vi "FGGA_Viewer_2.1.vi"() -> ()   [LabVIEW 2012]
uses:
  <vilib>/Utility/tcp.llb/UDP Multicast Read-Only Open.vi
  <vilib>/regexp/Match Regular Expression.xnode
panel:
  in  "Tab Control":enum32{"MAIN_DATA", "MONITORING"}(tab)
  out "FGGA":cluster{dbl, dbl, dbl}(graph)
  out "FGGA_Mon":cluster{dbl, dbl, dbl}(graph)
  out "Running?":bool
  in  "reset x-axis":bool
  out "error out":errorcluster
  in  "stop":bool
  out "data out":string
  in  "name":string="225.0.0.0"
  in  "Port":u16=50005
  # "CONCENTRATIONS ARE NOT ABSOLUTE"
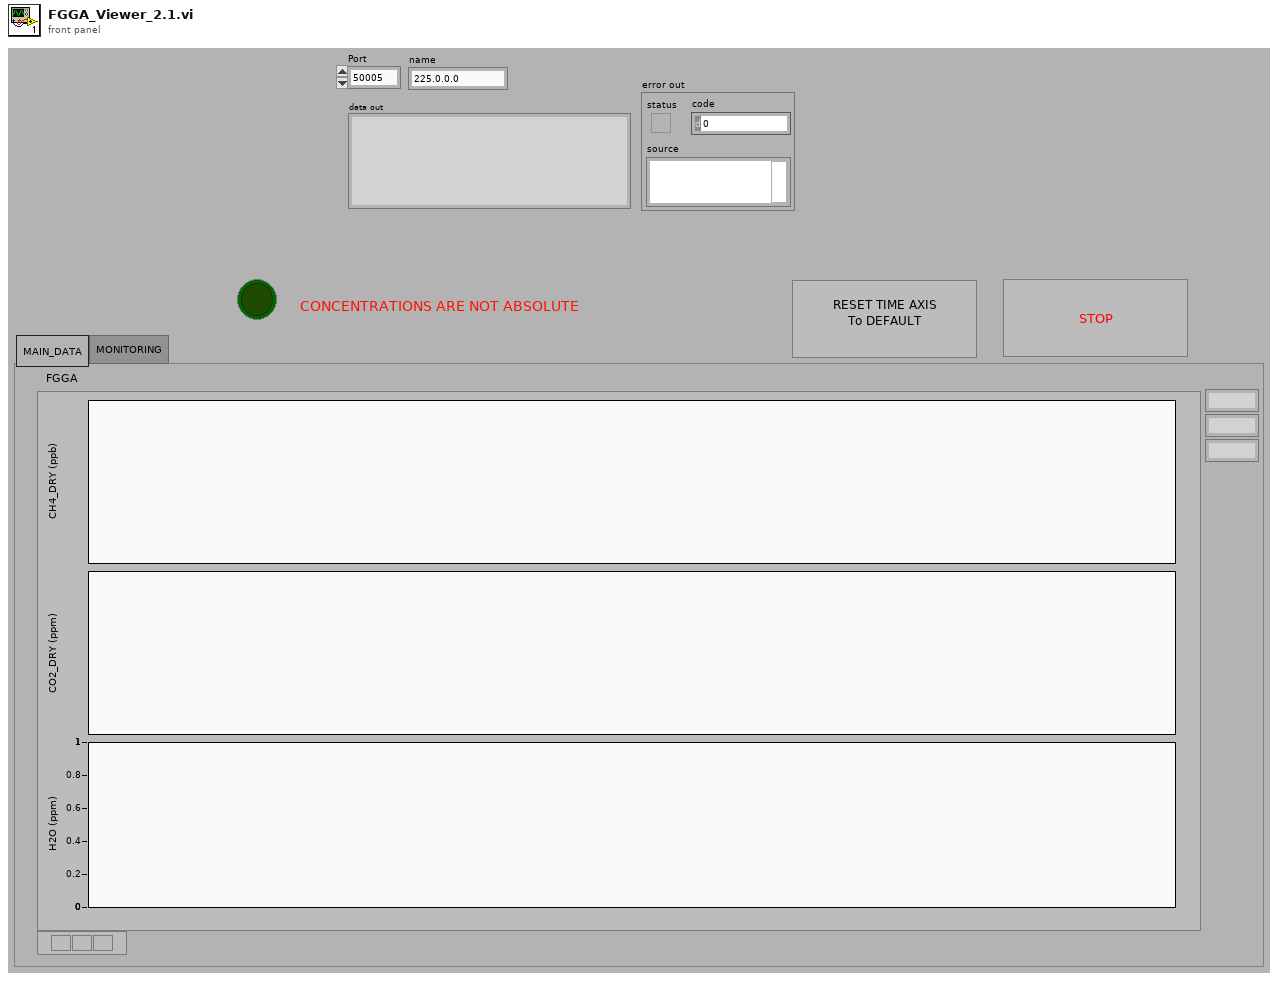
[diagram p1: front panel]
types:
  T1 = cluster{"[0]":i32, "[1]":i32, "[2]":i32, "[3]":i32, "[4]":i32, "[5]":i32, "[6]":i32, "[7]":i32, "[8]":i32}
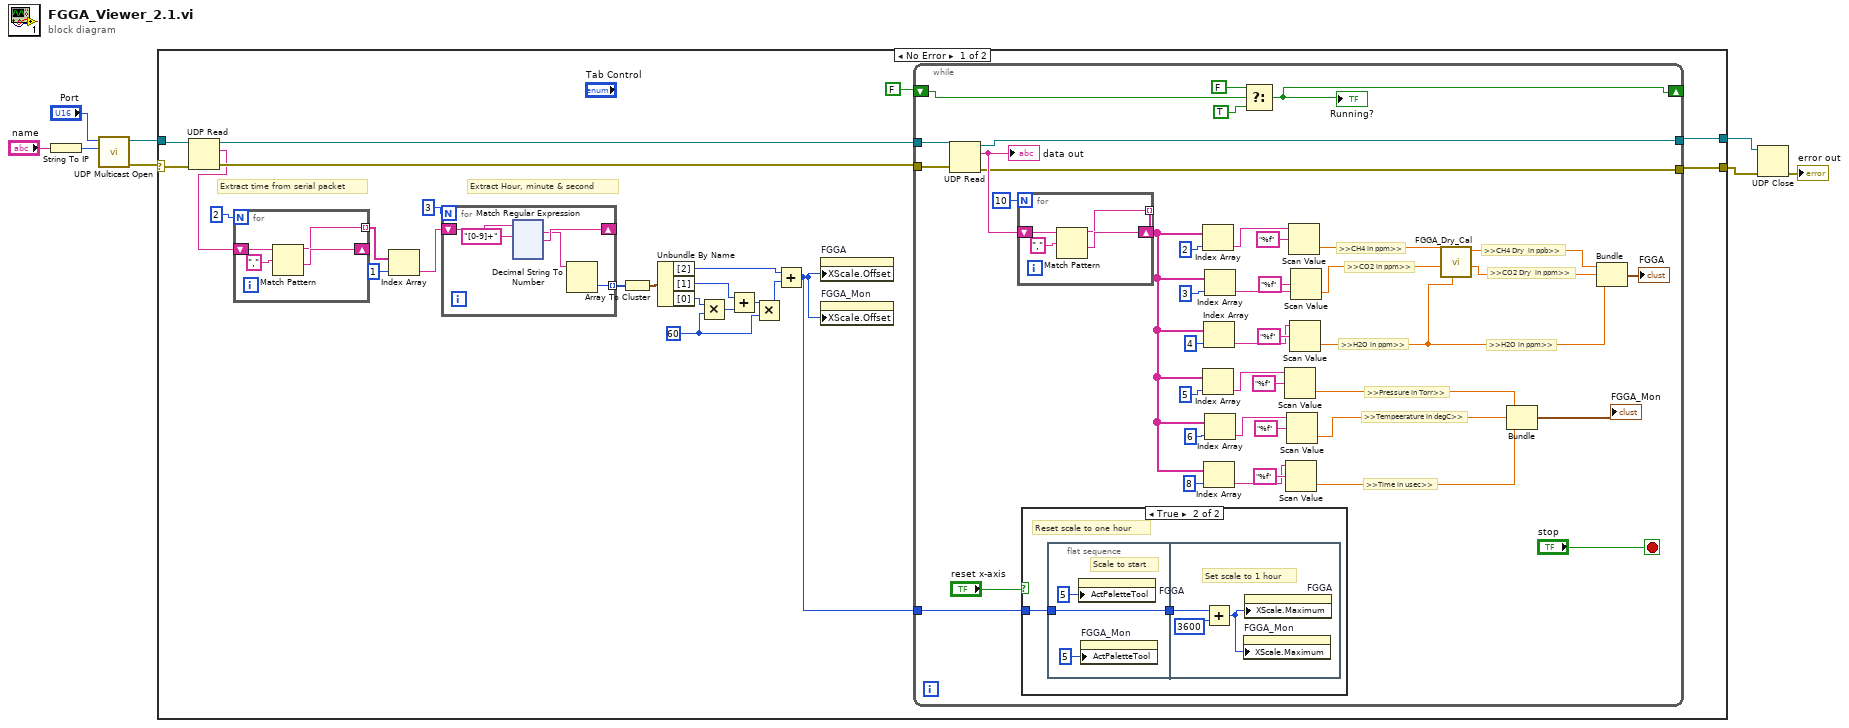
[diagram p0: block diagram]
diagram:
  n1 = String To IP(1:"name") -> (0:w7:u32)
  n2 = call-poly <vilib>:"UDP Multicast Open.vi"("multicast addr"=w7, "port"="Port") -> ("error out"=w4:errorcluster, "connection ID"=w5:refnum<k16>)  [unwired: 7 in, 1 out]
  n3 = case shown="No Error" w4 {
    selector: w4 -> [w29 w206]
    tunnel: w5 -> [w28 w207]
    tunnel: [w31 w206] -> w3
    tunnel: [w30 w207] -> w2
    frame No Error {
      w17 = 60
      # "Extract Hour, minute & second"
      # "Extract time from serial packet"
      n4 = UDP Read(connection ID=w28, 8:w29) -> (data out=w22:string, error out=w26:errorcluster, 3:w27:refnum<k16>)  [unwired: 2 in, 2 out]
      n5 = for {
        N: 2 -> [_]
        shift-right: [w150] -> _
        shift-left: w22 -> [w148]
        tunnel: [w149] -> w23 mode=indexing
        n6 = Match Pattern(string=w148, regular expression=",") -> (before substring=w149:string, after substring=w150:string)  [unwired: 1 in, 2 out]
      }
      n7 = Index Array(array=w23, index=1) -> (element=w18:string)
      n8 = for {
        N: 3 -> [_]
        tunnel: [w33] -> w20 mode=indexing
        shift-right: [w34] -> _
        shift-left: w18 -> [w35]
        n9 = xnode "Match Regular Expression"("input string"=w35, "regular expression"="[0-9]+") -> ("whole match"=w32:string, "after match"=w34:string)  [unwired: 4 in, 3 out]
        n10 = Decimal String To Number(string=w32) -> (number=w33:i32)  [unwired: 2 in, 1 out]
      }
      n11 = Array To Cluster(array=w20) -> (cluster=w19:T1)
      n12 = Unbundle By Name(w19) -> ("[2]"=w11:i32, "[1]"=w12:i32, "[0]"=w13:i32)
      n13 = Multiply(x=w13, y=w17) -> (x*y=w14:i32)
      n14 = Add(x=w12, y=w14) -> (x+y=w15:i32)
      n15 = Multiply(x=w15, y=w17) -> (x*y=w16:i32)
      n16 = Add(x=w11, y=w16) -> (x+y=w9:i32)
      n17 = property on="FGGA" class="WFChart (strict)"("XScale.Offset"=w9) -> ()  [unwired: 2 in, 2 out]
      n18 = property on="FGGA_Mon" class="WFChart (strict)"("XScale.Offset"=w9) -> ()  [unwired: 2 in, 2 out]
      n19 = while {
        tunnel: w27 -> [w193]
        tunnel: w26 -> [w192]
        tunnel: [w180] -> w31
        tunnel: [w178] -> w30
        tunnel: w9 -> [w175]
        shift-right: [w171] -> _
        shift-left: FALSE -> [w174]
        stop <- "stop" stop-if-true
        # ">>H2O in ppm>>"
        # ">>CO2 Dry  in ppm>>"
        # ">>CH4 Dry  in ppb>>"
        # ">>Time in usec>>"
        # ">>Tempeerature in degC>>"
        # ">>Pressure in Torr>>"
        # ">>H2O in ppm>>"
        # ">>CO2 in ppm>>"
        # ">>CH4 in ppm>>"
        n20 = UDP Read(connection ID=w193, 8:w192) -> (data out=w181:string, error out=w180:errorcluster, 3:w178:refnum<k16>)  [unwired: 2 in, 2 out]
        "data out" <- w181
        n21 = for {
          N: 10 -> [_]
          shift-right: [w204] -> _
          shift-left: w181 -> [w202]
          tunnel: [w203] -> w158 mode=indexing
          n22 = Match Pattern(string=w202, regular expression=",") -> (before substring=w203:string, after substring=w204:string)  [unwired: 1 in, 2 out]
        }
        n23 = case shown="True" "reset x-axis" {
          tunnel: w175 -> [_ w195]
          frame False {
          }
          frame True {
            # "Reset scale to one hour"
            n24 = flat-sequence {
              tunnel: w195 -> [w198]
              tunnel: [w198] -> w194
              tunnel: w194 -> [w201]
              frame #0 {
                # "Scale to start"
                n25 = property on="FGGA" class="WFChart (strict)"("ActPaletteTool"=5 ("Palette:Active Tool")) -> ()  [unwired: 2 in, 2 out]
                n26 = property on="FGGA_Mon" class="WFChart (strict)"("ActPaletteTool"=5 ("Palette:Active Tool")) -> ()  [unwired: 2 in, 2 out]
              }
              frame #1 {
                # "Set scale to 1 hour"
                n27 = Add(x=w201, y=3600) -> (x+y=w199:i32)
                n28 = property on="FGGA_Mon" class="WFChart (strict)"("XScale.Maximum"=w199) -> ()  [unwired: 2 in, 2 out]
                n29 = property on="FGGA" class="WFChart (strict)"("XScale.Maximum"=w199) -> ()  [unwired: 2 in, 2 out]
              }
            }
          }
        }
        n30 = Index Array(array=w158, index=2) -> (element=w189:string)
        n31 = Index Array(array=w158, index=5) -> (element=w169:string)
        n32 = Index Array(array=w158, index=4) -> (element=w182:string)
        n33 = Index Array(array=w158, index=8) -> (element=w162:string)
        n34 = Index Array(array=w158, index=3) -> (element=w186:string)
        n35 = Index Array(array=w158, index=6) -> (element=w166:string)
        n36 = Select(t=FALSE, s=w174, f=TRUE) -> (s? t:f=w171:bool)
        "Running?" <- w171
        n37 = Scan Value(string=w169, format string="%f") -> (value=w161:dbl)  [unwired: 1 in, 1 out]
        n38 = Scan Value(string=w162, format string="%f") -> (value=w159:dbl)  [unwired: 1 in, 1 out]
        n39 = Scan Value(string=w166, format string="%f") -> (value=w160:dbl)  [unwired: 1 in, 1 out]
        n40 = Scan Value(string=w189, format string="%f") -> (value=w156:dbl)  [unwired: 1 in, 1 out]
        n41 = Scan Value(string=w182, format string="%f") -> (value=w154:dbl)  [unwired: 1 in, 1 out]
        n42 = Scan Value(string=w186, format string="%f") -> (value=w155:dbl)  [unwired: 1 in, 1 out]
        n43 = call "FGGA_Dry_Cal.vi"("H2O"=w154, "CO2_Wet"=w155, "CH4_Wet"=w156) -> ("CO2_Dry"=w153:dbl, "CH4_Dry"=w152:dbl)  [unwired: 7 in]
        n44 = Bundle(w161, w160, w159) -> (→"FGGA_Mon":cluster{dbl, dbl, dbl})  [unwired: 1 in]
        n45 = Bundle("CH4_Dry"=w152, "CO2_Dry"=w153, w154) -> (→"FGGA":cluster{"CH4_Dry":dbl, "CO2_Dry":dbl, dbl})  [unwired: 1 in]
      }
    }
    frame Error {
    }
  }
  n46 = UDP Close(connection ID=w2, 8:w3) -> (error out=→"error out":errorcluster)  [unwired: 1 out]
